vi "compute_samplingrate_samples_NPLCmode.vi"(2 "Samplingrate":dbl, 3 "Nchannel":dbl, 4 "NPLC":dbl) -> (0 "effective samplingrate":dbl, 1 "samples to read":u32)   [LabVIEW 2013]
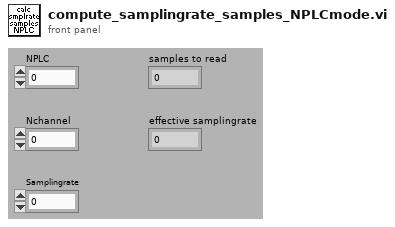
[diagram p1: front panel]
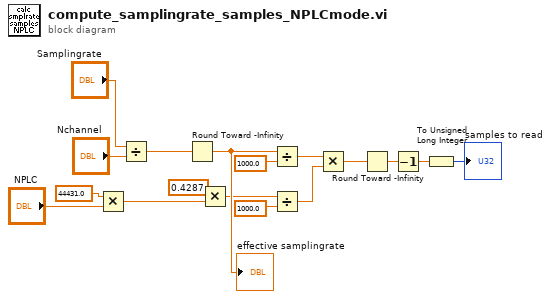
[diagram p0: block diagram]
diagram:
  n1 = Multiply(x=44431.0, y="NPLC") -> (x*y=w14:dbl)
  n2 = Divide(x="Samplingrate", y="Nchannel") -> (x/y=w1:dbl)
  n3 = Round Toward -Infinity(1:w1) -> (0:w11:dbl)
  "effective samplingrate" <- w11
  n4 = Multiply(x=0.4287, y=w14) -> (x*y=w5:dbl)
  n5 = Divide(x=w11, y=1000.0) -> (x/y=w12:dbl)
  n6 = Divide(x=w5, y=1000.0) -> (x/y=w9:dbl)
  n7 = Multiply(x=w12, y=w9) -> (x*y=w7:dbl)
  n8 = Round Toward -Infinity(1:w7) -> (0:w8:dbl)
  n9 = Decrement(x=w8) -> (x-1=w13:dbl)
  n10 = To Unsigned Long Integer(number=w13) -> (unsigned 32bit integer=→"samples to read":u32)
